vi "V3_IRCal_PID.vi"(7 "Direction":T1(ring)=enum."right", 8 "Error In":errorcluster) -> (0 "Error Out":errorcluster, 2 "Waveform Chart":T3(graph)={"Valtage[0]"=1.459096459096459, "Valtage[1]"=1.492063492063492, "Valtage[2]"=1.459096459096459})   [LabVIEW 2019]
uses:
  <vilib>/Platform/TimedLoop/XDataNode/timing_clust.ctl
  <vilib>/Platform/TimedLoop/XDataNode/nitl_modes.ctl
  <vilib>/Platform/TimedLoop/XDataNode/wakeup.ctl
  WSCbot_V3_Toolkit.lvlibp/WSCBOTV3_Toolkit/Sensor/LowLevel/IR_Chanel.ctl
  <vilib>/addons/control/pid/pid.llb/PID (DBL).vi
  <vilib>/platform/TimedLoop/XDataNode/XDataNode.xnode
  WSCbot_V3_Toolkit.lvlibp
  <vilib>/Platform/TimedLoop/XDataNode/XDNodeRunTimeDep.lvlib
  <vilib>/addons/control/pid/NI_PID_pid.lvlib
panel:
  in  "Y_distance(V)":dbl=1.5
  in  "X_distance(V)":dbl=1.5
  in  "return_error":dbl=0.03
  out "Boolean 3":bool=TRUE
  out "Boolean 2":bool=TRUE
  out "Boolean":bool=TRUE
  in  "Stop Button":bool
  in  "PID 左右":T2={"proportional gain (Kc)"=3.0, "integral time (Ti, min)"=0.0, "derivative time (Td, min)"=0.0001} {"derivative time (Td, min)" format="%#.6f"; "integral time (Ti, min)" format="%#.3f"; "proportional gain (Kc)" format="%#.3f"}
  in  "PID 自旋":T2={"proportional gain (Kc)"=4.5, "integral time (Ti, min)"=0.0, "derivative time (Td, min)"=0.0001} {"derivative time (Td, min)" format="%#.6f"; "integral time (Ti, min)" format="%#.3f"; "proportional gain (Kc)" format="%#.3f"}
  in  "PID 前後":T2={"proportional gain (Kc)"=1.5, "integral time (Ti, min)"=0.0, "derivative time (Td, min)"=0.0001} {"derivative time (Td, min)" format="%#.6f"; "integral time (Ti, min)" format="%#.3f"; "proportional gain (Kc)" format="%#.3f"}
  out "Spend time":dbl=5.445
  out "Waveform Chart 2":T3(graph)={"Valtage[0]"=0.04090354090354098, "Valtage[1]"=-0.03296703296703307, "Valtage[2]"=0.007936507936507908}
  out "result":bool=TRUE
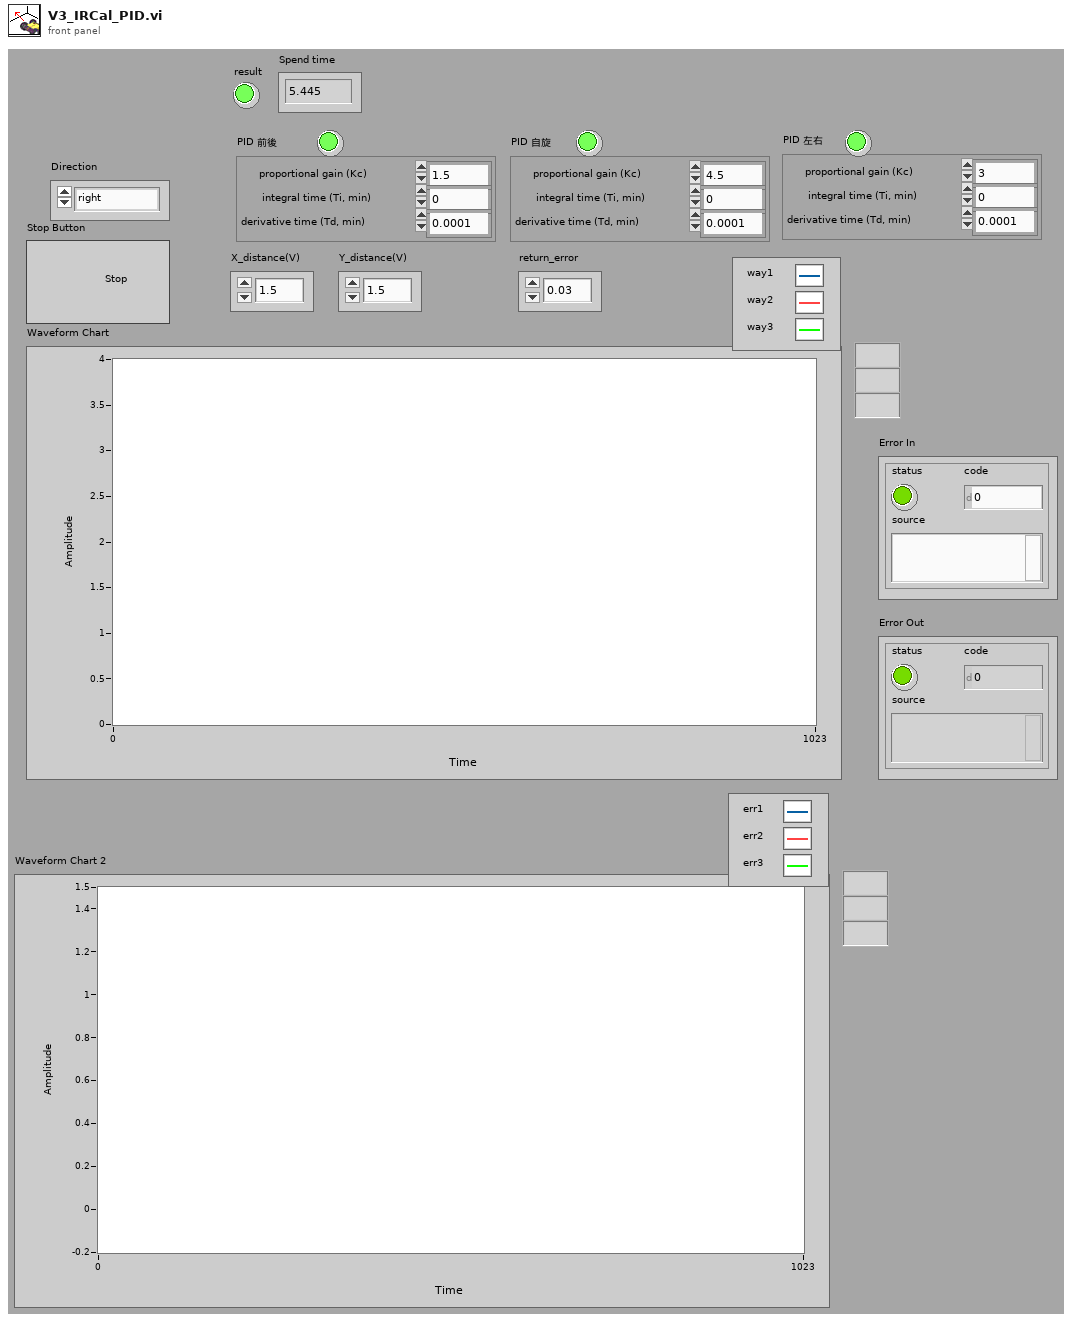
[diagram p1: front panel]
types:
  T1 = enum16{"Right_up", "Right_down", "Left_down", "Left_up", "left", "right", "up", "down"}
  T2 = cluster{"proportional gain (Kc)":dbl, "integral time (Ti, min)":dbl, "derivative time (Td, min)":dbl}
  T3 = cluster{"Valtage[0]":dbl, "Valtage[1]":dbl, "Valtage[2]":dbl}
  T4 = typedef "XDNodeRunTimeDep.lvlib/timing_clust.ctl" = cluster{"Expected End [f-1]":u64, "Actual End [f-1]":u64, "Finished Late? [f-1]":bool, "Expected End [i-1]":u64, "Actual End [i-1]":u64, "Finished Late? [i-1]":bool, "Expected Start [i]":u64, "Actual Start [i]":u64, "Expected Start [f]":u64, "Actual Start [f]":u64, "Source Name":string, "Structure Name":string, "Period":i64, "Deadline":i64, "Offset":i64, "Start":i64, "Priority":i32, "Timeout":i32, "Mode":T5, "Wakeup Reason":T6, "Error":errorcluster, "Source Type":string, "Secondary Source Type":string, "Global End Time":u64, "Global Start Time":u64, "Frame Duration":u64, "Iteration Duration":u64, "Assigned CPU":i32, "I/O Scan Engine Mode":u32}
  T5 = typedef "XDNodeRunTimeDep.lvlib/nitl_modes.ctl" = enum32{"No Change", "Process missed periods, maintain original phase", "Discard missed periods, maintain original phase", "Process missed periods, ignore original phase", "Discard missed periods, ignore original phase"}
  T6 = typedef "XDNodeRunTimeDep.lvlib/wakeup.ctl" = enum32{"Normal", "Aborted", "Asynchronous wakeup", "Timing source error", "Timed loop error", "Timeout"}
  T7 = typedef "WSCbot_V3_Toolkit.lvlibp/IR_Chanel.ctl" = enum16{"IR_LF", "IR_LB", "IR_BL", "IR_BR", "IR_RB", "IR_RF", "IR_FR", "IR_FL"}
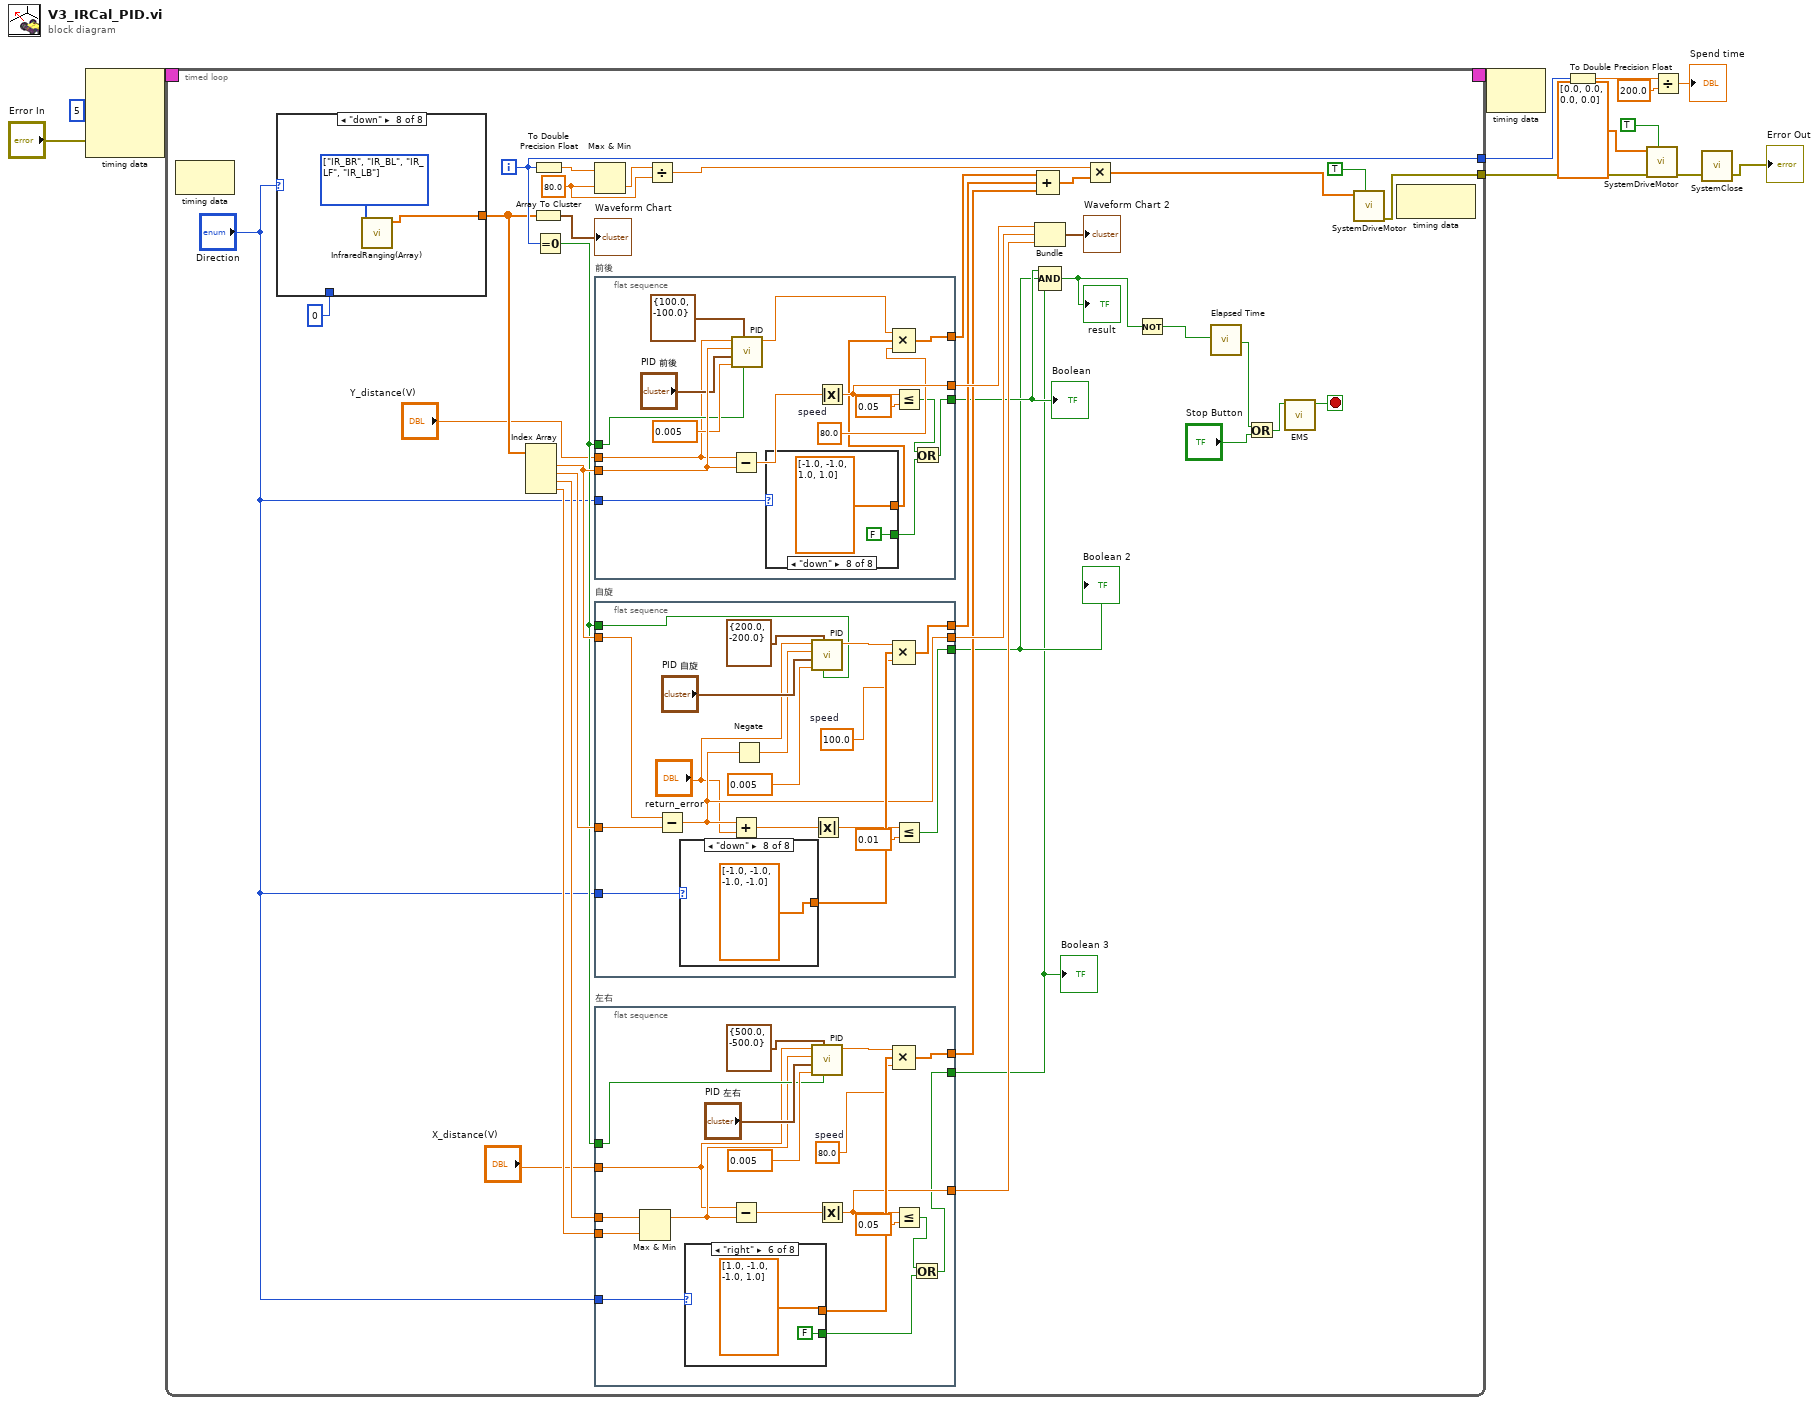
[diagram p0: block diagram]
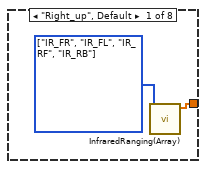
[diagram p2: hidden frame]
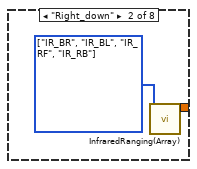
[diagram p3: hidden frame]
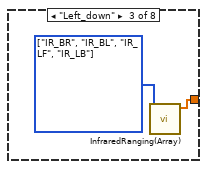
[diagram p4: hidden frame]
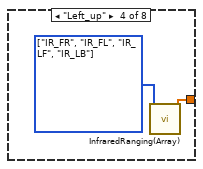
[diagram p5: hidden frame]
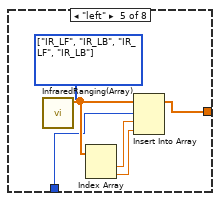
[diagram p6: hidden frame]
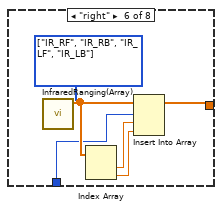
[diagram p7: hidden frame]
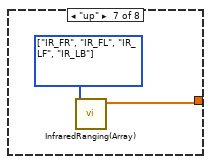
[diagram p8: hidden frame]
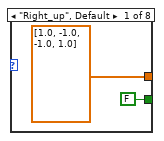
[diagram p9: hidden frame]
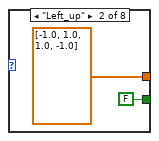
[diagram p10: hidden frame]
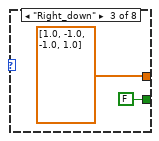
[diagram p11: hidden frame]
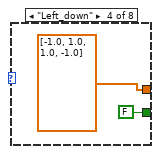
[diagram p12: hidden frame]
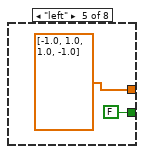
[diagram p13: hidden frame]
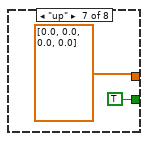
[diagram p14: hidden frame]
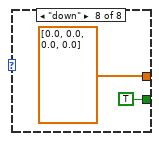
[diagram p15: hidden frame]
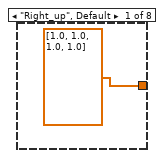
[diagram p16: hidden frame]
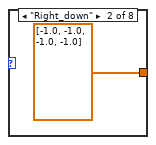
[diagram p17: hidden frame]
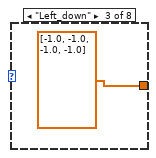
[diagram p18: hidden frame]
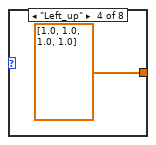
[diagram p19: hidden frame]
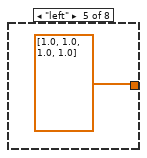
[diagram p20: hidden frame]
diagram:
  n1 = node-c288(i64 5 ("Period"), "Error In") -> (w13:T4)  [unwired: 2 in]
  n2 = timed-loop {
    timing: w13 -> [_]
    timing-out: [_] -> w12
    tunnel: [w44] -> w10
    tunnel: [w30] -> w6
    i -> [w30]
    stop <- w35 stop-if-true
    w39 = 80.0 ("y")
    n3 = node-c288() -> ()  [unwired: 1 in, 1 out]
    n4 = case shown="\"down\"" "Direction" {
      tunnel: [w50 w52 w54 w56 w59 w65 w70 w72] -> w18
      tunnel: 0 ("index") -> [_ _ _ _ w58 w64 _ _]
      frame "Right_up", Default {
        w51 = T7[] [enum."IR_FR", enum."IR_FL", enum."IR_RF", enum."IR_RB"] items=["IR_LF", "IR_LB", "IR_BL", "IR_BR", "IR_RB", "IR_RF", "IR_FR", "IR_FL"] ("IR_Chanel")
        n5 = call "InfraredRanging(Array).vi"("IR_Chanel"=w51) -> ("Valtage"=w50:dbl[])  [unwired: 9 in, 1 out]
      }
      frame "Right_down" {
        w53 = T7[] [enum."IR_BR", enum."IR_BL", enum."IR_RF", enum."IR_RB"] items=["IR_LF", "IR_LB", "IR_BL", "IR_BR", "IR_RB", "IR_RF", "IR_FR", "IR_FL"] ("IR_Chanel")
        n6 = call "InfraredRanging(Array).vi"("IR_Chanel"=w53) -> ("Valtage"=w52:dbl[])  [unwired: 9 in, 1 out]
      }
      frame "Left_down" {
        w55 = T7[] [enum."IR_BR", enum."IR_BL", enum."IR_LF", enum."IR_LB"] items=["IR_LF", "IR_LB", "IR_BL", "IR_BR", "IR_RB", "IR_RF", "IR_FR", "IR_FL"] ("IR_Chanel")
        n7 = call "InfraredRanging(Array).vi"("IR_Chanel"=w55) -> ("Valtage"=w54:dbl[])  [unwired: 9 in, 1 out]
      }
      frame "Left_up" {
        w57 = T7[] [enum."IR_FR", enum."IR_FL", enum."IR_LF", enum."IR_LB"] items=["IR_LF", "IR_LB", "IR_BL", "IR_BR", "IR_RB", "IR_RF", "IR_FR", "IR_FL"] ("IR_Chanel")
        n8 = call "InfraredRanging(Array).vi"("IR_Chanel"=w57) -> ("Valtage"=w56:dbl[])  [unwired: 9 in, 1 out]
      }
      frame "left" {
        w60 = T7[] [enum."IR_LF", enum."IR_LB", enum."IR_LF", enum."IR_LB"] items=["IR_LF", "IR_LB", "IR_BL", "IR_BR", "IR_RB", "IR_RF", "IR_FR", "IR_FL"] ("IR_Chanel")
        n9 = call "InfraredRanging(Array).vi"("IR_Chanel"=w60) -> ("Valtage"=w63:dbl[])  [unwired: 9 in, 1 out]
        n10 = Index Array(array=w63) -> (element #1=w61:dbl, element #2=w62:dbl)  [unwired: 2 in]
        n11 = Insert Into Array(array=w63, index=w58, new element #1=w61, new element #2=w62) -> (w59:dbl[])
      }
      frame "right" {
        w66 = T7[] [enum."IR_RF", enum."IR_RB", enum."IR_LF", enum."IR_LB"] items=["IR_LF", "IR_LB", "IR_BL", "IR_BR", "IR_RB", "IR_RF", "IR_FR", "IR_FL"] ("IR_Chanel")
        n12 = call "InfraredRanging(Array).vi"("IR_Chanel"=w66) -> ("Valtage"=w69:dbl[])  [unwired: 9 in, 1 out]
        n13 = Index Array(array=w69) -> (element #1=w67:dbl, element #2=w68:dbl)  [unwired: 2 in]
        n14 = Insert Into Array(array=w69, index=w64, new element #1=w67, new element #2=w68) -> (w65:dbl[])
      }
      frame "up" {
        w71 = T7[] [enum."IR_FR", enum."IR_FL", enum."IR_LF", enum."IR_LB"] items=["IR_LF", "IR_LB", "IR_BL", "IR_BR", "IR_RB", "IR_RF", "IR_FR", "IR_FL"] ("IR_Chanel")
        n15 = call "InfraredRanging(Array).vi"("IR_Chanel"=w71) -> ("Valtage"=w70:dbl[])  [unwired: 9 in, 1 out]
      }
      frame "down" {
        w73 = T7[] [enum."IR_BR", enum."IR_BL", enum."IR_LF", enum."IR_LB"] items=["IR_LF", "IR_LB", "IR_BL", "IR_BR", "IR_RB", "IR_RF", "IR_FR", "IR_FL"] ("IR_Chanel")
        n16 = call "InfraredRanging(Array).vi"("IR_Chanel"=w73) -> ("Valtage"=w72:dbl[])  [unwired: 9 in, 1 out]
      }
    }
    n17 = Index Array(array=w18) -> (element #1=w46:dbl, element #2=w48:dbl, element #3=w47:dbl, element #4=w22:dbl)  [unwired: 4 in]
    n18 = Array To Cluster(array=w18) -> (cluster=→"Waveform Chart":T3)
    n19 = To Double Precision Float(number=w30) -> (double precision float=w41:dbl)
    n20 = Equal To 0?(x=w30) -> (x = 0?=w29:bool)
    n21 = Max & Min(x=w41, y=w39) -> (min(x,y)=w40:dbl)  [unwired: 1 out]
    n22 = flat-sequence "前後" {
      tunnel: w46 -> [w149]
      tunnel: [w142] -> w28
      tunnel: [w143] -> w33
      tunnel: w29 -> [w144]
      tunnel: [w135] -> w25
      tunnel: "Direction" -> [w140]
      tunnel: "Y_distance(V)" -> [w138]
      frame #0 {
        w141 = 80.0  # speed
        n23 = Subtract(x=w138, y=w149) -> (x-y=w150:dbl)
        n24 = call-poly <vilib>:"PID.vi"("reinitialize? (F)"=w144, "output range"=cluster{"output high":dbl, "output low":dbl} {"output high"=100.0, "output low"=-100.0}, "dt (s)"=0.005, "PID gains"="PID 前後", "process variable"=w149, "setpoint"=w138) -> ("output"=w145:dbl)  [unwired: 4 in, 1 out]
        n25 = case shown="\"down\"" w140 {
          tunnel: [dbl[] [1.0, 1.0, -1.0, -1.0] ("y") dbl[] [-1.0, -1.0, 1.0, 1.0] ("y") dbl[] [-1.0, -1.0, 1.0, 1.0] ("y") dbl[] [1.0, 1.0, -1.0, -1.0] ("y") dbl[] [0.0, 0.0, 0.0, 0.0] ("y") dbl[] [0.0, 0.0, 0.0, 0.0] ("y") dbl[] [1.0, 1.0, -1.0, -1.0] ("y") dbl[] [-1.0, -1.0, 1.0, 1.0] ("y")] -> w139
          tunnel: [FALSE FALSE FALSE FALSE TRUE TRUE FALSE FALSE] -> w136
          frame "Right_up", Default {
          }
          frame "Left_down" {
          }
          frame "Right_down" {
          }
          frame "Left_up" {
          }
          frame "left" {
          }
          frame "right" {
          }
          frame "up" {
          }
          frame "down" {
          }
        }
        n26 = Absolute Value(x=w150) -> (abs(x)=w143:dbl)
        n27 = Compound Arithmetic op=MULTIPLY(w145, w139, w141) -> (w142:dbl[])
        n28 = Less Or Equal?(x=w143, y=0.05) -> (x <= y?=w137:bool)
        n29 = Or(x=w137, y=w136) -> (x .or. y?=w135:bool)
      }
    }
    n30 = flat-sequence "自旋" {
      tunnel: w48 -> [w126]
      tunnel: w46 -> [w119]
      tunnel: [w124] -> w27
      tunnel: [w122] -> w24
      tunnel: [w114] -> w32
      tunnel: w29 -> [w116]
      tunnel: "Direction" -> [w110]
      frame #0 {
        w111 = 100.0  # speed
        n31 = Subtract(x=w119, y=w126) -> (x-y=w114:dbl)
        n32 = case shown="\"down\"" w110 {
          tunnel: [dbl[] [1.0, 1.0, 1.0, 1.0] ("y") dbl[] [-1.0, -1.0, -1.0, -1.0] ("y") dbl[] [-1.0, -1.0, -1.0, -1.0] ("y") dbl[] [1.0, 1.0, 1.0, 1.0] ("y") dbl[] [1.0, 1.0, 1.0, 1.0] ("y") dbl[] [-1.0, -1.0, -1.0, -1.0] ("y") dbl[] [1.0, 1.0, 1.0, 1.0] ("y") dbl[] [-1.0, -1.0, -1.0, -1.0] ("y")] -> w125
          frame "Right_up", Default {
          }
          frame "Right_down" {
          }
          frame "Left_down" {
          }
          frame "Left_up" {
          }
          frame "left" {
          }
          frame "right" {
          }
          frame "up" {
          }
          frame "down" {
          }
        }
        n33 = Add(x=w114, y="return_error") -> (x+y=w113:dbl)
        n34 = Negate(x=w114) -> (-x=w115:dbl)
        n35 = call-poly <vilib>:"PID.vi"("reinitialize? (F)"=w116, "output range"=cluster{"output high":dbl, "output low":dbl} {"output high"=200.0, "output low"=-200.0}, "dt (s)"=0.005, "PID gains"="PID 自旋", "process variable"=w115, "setpoint"="return_error") -> ("output"=w118:dbl)  [unwired: 4 in, 1 out]
        n36 = Absolute Value(x=w113) -> (abs(x)=w112:dbl)
        n37 = Compound Arithmetic op=MULTIPLY(w118, w125, w111) -> (w124:dbl[])
        n38 = Less Or Equal?(x=w112, y=0.01) -> (x <= y?=w122:bool)
      }
    }
    n39 = flat-sequence "左右" {
      tunnel: w47 -> [w82]
      tunnel: [w91] -> w26
      tunnel: [w75] -> w23
      tunnel: [w83] -> w31
      tunnel: w29 -> [w85]
      tunnel: w22 -> [w81]
      tunnel: "Direction" -> [w78]
      tunnel: "X_distance(V)" -> [w77]
      frame #0 {
        w79 = 80.0  # speed
        n40 = Max & Min(x=w82, y=w81) -> (max(x,y)=w80:dbl)  [unwired: 1 out]
        n41 = case shown="\"right\"" w78 {
          tunnel: [dbl[] [1.0, -1.0, -1.0, 1.0] ("y") dbl[] [-1.0, 1.0, 1.0, -1.0] ("y") dbl[] [1.0, -1.0, -1.0, 1.0] ("y") dbl[] [-1.0, 1.0, 1.0, -1.0] ("y") dbl[] [-1.0, 1.0, 1.0, -1.0] ("y") dbl[] [1.0, -1.0, -1.0, 1.0] ("y") dbl[] [0.0, 0.0, 0.0, 0.0] ("y") dbl[] [0.0, 0.0, 0.0, 0.0] ("y")] -> w92
          tunnel: [FALSE FALSE FALSE FALSE FALSE FALSE TRUE TRUE] -> w74
          frame "Right_up", Default {
          }
          frame "Left_up" {
          }
          frame "Right_down" {
          }
          frame "Left_down" {
          }
          frame "left" {
          }
          frame "right" {
          }
          frame "up" {
          }
          frame "down" {
          }
        }
        n42 = Subtract(x=w77, y=w80) -> (x-y=w89:dbl)
        n43 = call-poly <vilib>:"PID.vi"("reinitialize? (F)"=w85, "output range"=cluster{"output high":dbl, "output low":dbl} {"output high"=500.0, "output low"=-500.0}, "dt (s)"=0.005, "PID gains"="PID 左右", "process variable"=w80, "setpoint"=w77) -> ("output"=w84:dbl)  [unwired: 4 in, 1 out]
        n44 = Absolute Value(x=w89) -> (abs(x)=w83:dbl)
        n45 = Compound Arithmetic op=MULTIPLY(w84, w92, w79) -> (w91:dbl[])
        n46 = Less Or Equal?(x=w83, y=0.05) -> (x <= y?=w76:bool)
        n47 = Or(x=w76, y=w74) -> (x .or. y?=w75:bool)
      }
    }
    n48 = Divide(x=w40, y=w39) -> (x/y=w38:dbl)
    n49 = Bundle(w33, w32, w31) -> (→"Waveform Chart 2":cluster{dbl, dbl, dbl})  [unwired: 1 in]
    n50 = Compound Arithmetic op=ADD(w28, w27, w26) -> (w43:dbl[])
    n51 = Compound Arithmetic op=AND(w25, w24, w23) -> (w37:bool)
    "result" <- w37
    n52 = Multiply(x=w38, y=w43) -> (x*y=w42:dbl[])
    n53 = Not(x=w37) -> (.not. x?=w36:bool)
    n54 = call "Elapsed Time"("Reset"=w36) -> ("Time has Elapsed"=w20:bool)  [unwired: 11 in, 7 out]
    n55 = Or(x=w20, y="Stop Button") -> (x .or. y?=w19:bool)
    n56 = call "EMS.vi"("ProgramStop"=w19) -> ("EMS"=w35:bool)  [unwired: 9 in, 1 out]
    n57 = call "SystemDriveMotor.vi"("Enable?"=TRUE, "4xMotor(deg/s)"=w42) -> ("error out"=w44:errorcluster)  [unwired: 8 in, 1 out]
    n58 = node-c288() -> ()  [unwired: 1 in, 1 out]
    "Boolean" <- w25
    "Boolean 2" <- w24
    "Boolean 3" <- w23
  }
  n59 = node-c288(w12) -> ()  [unwired: 1 out]
  n60 = To Double Precision Float(number=w6) -> (double precision float=w5:dbl)
  n61 = call "SystemDriveMotor.vi"("Enable?"=TRUE, "error in"=w10, "4xMotor(deg/s)"=dbl[] [0.0, 0.0, 0.0, 0.0]) -> ("error out"=w7:errorcluster)  [unwired: 7 in, 1 out]
  n62 = Divide(x=w5, y=200.0) -> (x/y=→"Spend time":dbl)
  n63 = call "SystemClose.vi"("error in"=w7) -> ("error out"=→"Error Out":errorcluster)  [unwired: 2 in]
